vi "Polling Core.vi"(8 "Error In":errorcluster, 11 "CS++ObjectManager in":refnum<class "CS++ObjectManager.lvclass">) -> (0 "Error Out":errorcluster, 3 "CS++ObjectManager out":refnum<class "CS++ObjectManager.lvclass">)   [LabVIEW 2016, in "CS++ObjectManager.lvlib" / "CS++ObjectManager.lvclass"]
uses:
  CS++ObjectManager.lvclass
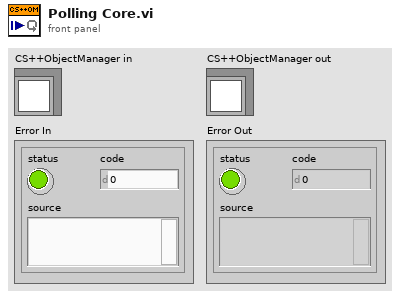
[diagram p1: front panel]
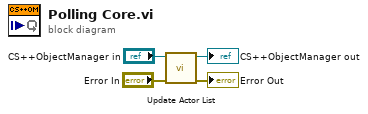
[diagram p0: block diagram]
diagram:
  n1 = call "Update Actor List.vi"("Error In"="Error In", "CS++ObjectManager in"="CS++ObjectManager in") -> ("Error Out"=→"Error Out":errorcluster, "CS++ObjectManager out"=→"CS++ObjectManager out":refnum<class "CS++ObjectManager.lvclass">)  [unwired: 8 in]
